vi "CRYGet Tree Step Type.vi"(0 "SequenceTree":refnum<vi>, 11 "Active Item Tag":string) -> (4 "reference out":refnum<vi>, 15 "Active Cell String3":string)   [LabVIEW 2013]
panel:
  in  "error in (no error)":errorcluster
  out "error out":errorcluster
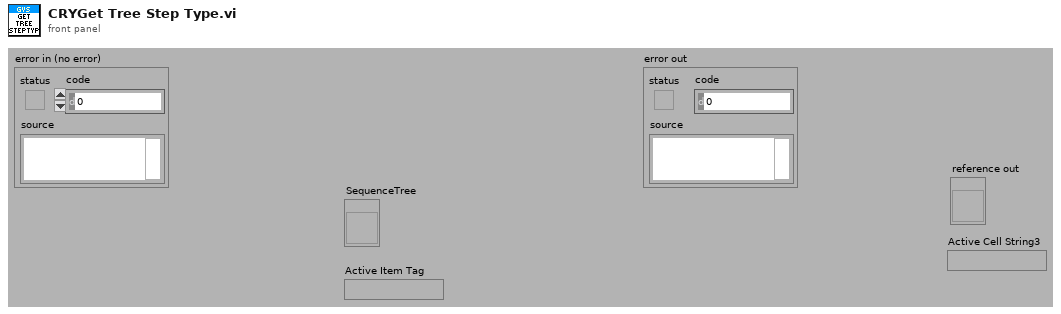
[diagram p1: front panel]
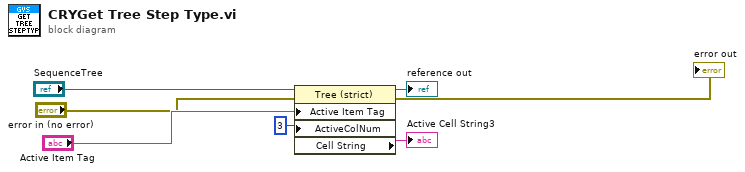
[diagram p0: block diagram]
diagram:
  n1 = property class="Tree (strict)"(reference="SequenceTree", error in="error in (no error)", "Active Item Tag"="Active Item Tag", "ActiveColNum"=3 ("Active Cell:Active Column Number")) -> (reference out=→"reference out":refnum<vi>, error out=→"error out":errorcluster, "Cell String"=→"Active Cell String3":string)
